vi "demo_2 Continuous Run.vi"() -> ()   [LabVIEW 2020]
panel:
  out "circSts":bool
  in  "bExit":bool
  in  "bStop":bool
  in  "bStart":bool
  in  "microstepping":u16(ring)=32 caption="细分" items=["1 (200)"=1, "2 (400)"=2, "4 (800)"=4, "8 (1600)"=8, "16 (3200)"=16, "32 (6400)"=32]
  in  "speed":u16 caption="转速 (RPM)"
  in  "direction":u16(ring) caption="旋向" items=["positive", "negative"]
  in  "VISA resource name":refnum<visa-resource-name> caption="VISA资源"
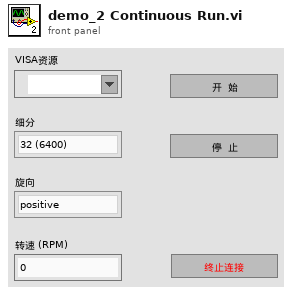
[diagram p1: front panel]
types:
  T1 = cluster{"full step angle":dbl, "microstepping":u16, "start frequency":u16, "stop frequency":u16, "screw pitch":dbl, "distance":dbl, "stop mode":u16, "direction":u16, "speed":u16, "relative / absolute":u16}
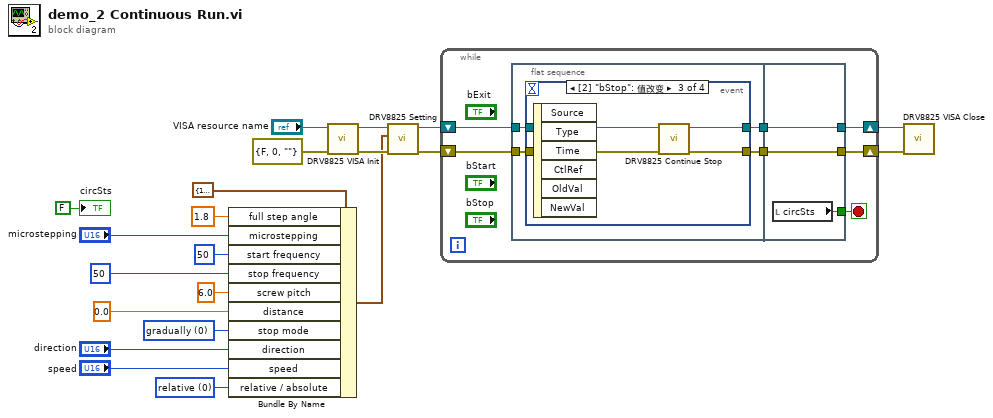
[diagram p0: block diagram]
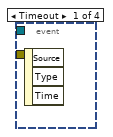
[diagram p2: hidden frame]
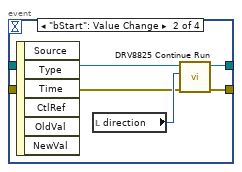
[diagram p3: hidden frame]
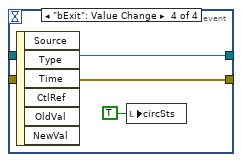
[diagram p4: hidden frame]
diagram:
  w13 = u16 0 items=["gradually", "immediately"] ("stop mode")
  w12 = u16 0 items=["relative", "absolute"] ("relative / absolute")
  n1 = Bundle By Name(cluster=T1 {"full step angle"=1.8, "microstepping"=32, "start frequency"=50, "stop frequency"=50, "screw pitch"=360.0, "distance"=0.0, "stop mode"=0, "direction"=0, "speed"=50, "relative / absolute"=0} ("settings"), "full step angle"=1.8, "microstepping"="microstepping", "start frequency"=u16 50, "stop frequency"=u16 50, "screw pitch"=6.0, "distance"=0.0, "stop mode"=w13, "direction"="direction", "speed"="speed", "relative / absolute"=w12) -> (w7:T1)
  n2 = call "DRV8825 VISA Init.vi"("error in (no error)"=errorcluster {"status"=FALSE, "code"=0, "source"=""}, "VISA resource name"="VISA resource name") -> ("error out"=w18:errorcluster, "VISA resource name out"=w19:refnum<visa-resource-name>)  [unwired: 8 in]
  n3 = call "DRV8825 Setting.vi"("error in (no error)"=w18, "settings"=w7, "VISA resource name"=w19) -> ("error out"=w4:errorcluster, "VISA resource name out"=w5:refnum<visa-resource-name>)  [unwired: 7 in]
  n4 = while {
    shift-right: [w26] -> w3
    shift-left: w5 -> [w28]
    shift-right: [w25] -> w2
    shift-left: w4 -> [w27]
    stop <- w22 stop-if-true
    n5 = flat-sequence {
      tunnel: w28 -> [w32]
      tunnel: w27 -> [w31]
      tunnel: [w30] -> w24
      tunnel: [w29] -> w23
      tunnel: [w46] -> w25
      tunnel: [w47] -> w26
      tunnel: w24 -> [w47]
      tunnel: w23 -> [w46]
      tunnel: [w45] -> w22
      frame #0 {
        n6 = event shown="[2] \"bStop\": 值改变" {
          selector: _ -> [_ _ _ _]
          dyn-events: _ -> [_ _ _ _]
          timeout: _ -> [_ _ _ _]
          tunnel: w32 -> [_ w37 w41 w43]
          tunnel: w31 -> [_ w35 w40 w42]
          tunnel: [_ w34 w39 w43] -> w30
          tunnel: [_ w33 w38 w42] -> w29
          event Timeout {
            n7 = event-data() -> ()  [unwired: 1 in, 3 out]
          }
          event "bStart": Value Change {
            n8 = event-data() -> ()  [unwired: 1 in, 6 out]
            n9 = local read "direction"() -> (w36:u16)
            n10 = call "DRV8825 Continue Run.vi"("error in (no error)"=w35, "direction"=w36, "VISA resource name"=w37) -> ("error out"=w33:errorcluster, "VISA resource name out"=w34:refnum<visa-resource-name>)  [unwired: 7 in]
          }
          event "bStop": Value Change {
            n11 = event-data() -> ()  [unwired: 1 in, 6 out]
            n12 = call "DRV8825 Continue Stop.vi"("error in (no error)"=w40, "VISA resource name"=w41) -> ("error out"=w38:errorcluster, "VISA resource name out"=w39:refnum<visa-resource-name>)  [unwired: 8 in]
          }
          event "bExit": Value Change {
            n13 = event-data() -> ()  [unwired: 1 in, 6 out]
            n14 = local write "circSts"(TRUE ("circSts")) -> ()
          }
        }
      }
      frame #1 {
        n15 = local read "circSts"() -> (w45:bool)
      }
    }
  }
  n16 = call "DRV8825 VISA Close.vi"("error in (no error)"=w2, "VISA resource name"=w3) -> ()  [unwired: 9 in, 1 out]
  "circSts" <- FALSE ("circSts")
